vi "FlatToRichnixnet_grpc_CreateSessionRequest.vi"(5 "OutputClusterType":T1, 11 "InputCluster":T3) -> (3 "OutputCluster":T1)   [LabVIEW 2025, in "grpc-xnet_client.lvlib"]
uses:
  nixnet_grpc_CreateSessionRequest_Flat.ctl
  nixnet_grpc_CreateSessionMode.ctl
  nidevice_grpc_SessionInitializationBehavior.ctl
  nixnet_grpc_CreateSessionRequest.ctl
  nixnet_grpc_CreateSessionRequest_mode_enum/nixnet_grpc_CreateSessionRequest_mode_enum.lvclass
  grpc-xnet_client.lvlib
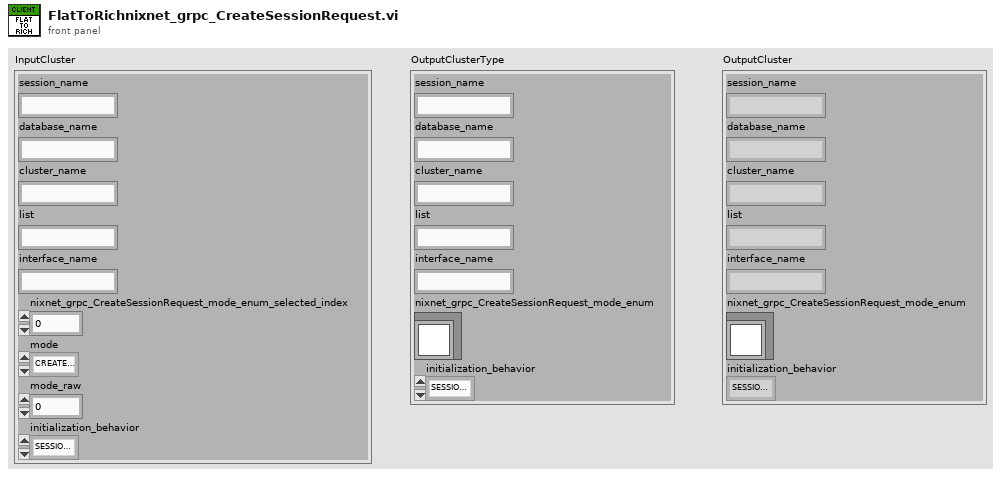
[diagram p1: front panel]
types:
  T1 = typedef "grpc-xnet_client.lvlib/nixnet_grpc_CreateSessionRequest.ctl" = cluster{"session_name":string, "database_name":string, "cluster_name":string, "list":string, "interface_name":string, "nixnet_grpc_CreateSessionRequest_mode_enum":refnum<class "nixnet_grpc_CreateSessionRequest_mode_enum.lvclass">, "initialization_behavior":T2}
  T2 = typedef "grpc-xnet_client.lvlib/nidevice_grpc_SessionInitializationBehavior.ctl" = enum32{"SESSION_INITIALIZATION_BEHAVIOR_UNSPECIFIED", "SESSION_INITIALIZATION_BEHAVIOR_INITIALIZE_NEW", "SESSION_INITIALIZATION_BEHAVIOR_ATTACH_TO_EXISTING"}
  T3 = typedef "grpc-xnet_client.lvlib/nixnet_grpc_CreateSessionRequest_Flat.ctl" = cluster{"session_name":string, "database_name":string, "cluster_name":string, "list":string, "interface_name":string, "nixnet_grpc_CreateSessionRequest_mode_enum_selected_index":i32, "mode":T4, "mode_raw":u32, "initialization_behavior":T2}
  T4 = typedef "grpc-xnet_client.lvlib/nixnet_grpc_CreateSessionMode.ctl" = enum32{"CREATE_SESSION_MODE_SIGNAL_IN_SINGLE_POINT", "CREATE_SESSION_MODE_SIGNAL_IN_WAVEFORM", "CREATE_SESSION_MODE_SIGNAL_IN_XY", "CREATE_SESSION_MODE_SIGNAL_OUT_SINGLE_POINT", "CREATE_SESSION_MODE_SIGNAL_OUT_WAVEFORM", "CREATE_SESSION_MODE_SIGNAL_OUT_XY", "CREATE_SESSION_MODE_FRAME_IN_STREAM", "CREATE_SESSION_MODE_FRAME_IN_QUEUED", "CREATE_SESSION_MODE_FRAME_IN_SINGLE_POINT", "CREATE_SESSION_MODE_FRAME_OUT_STREAM", "CREATE_SESSION_MODE_FRAME_OUT_QUEUED", "CREATE_SESSION_MODE_FRAME_OUT_SINGLE_POINT", "CREATE_SESSION_MODE_SIGNAL_CONVERSION_SINGLE_POINT"}
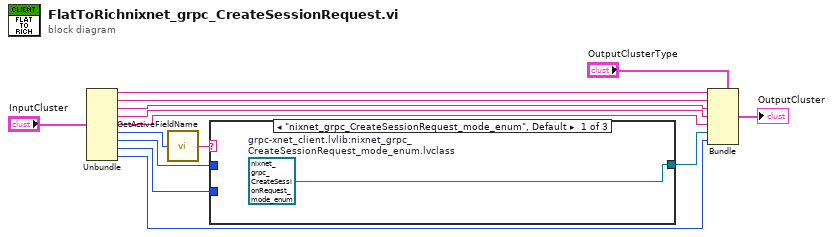
[diagram p0: block diagram]
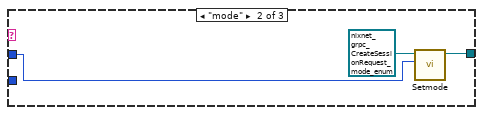
[diagram p2: hidden frame]
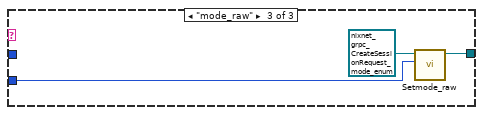
[diagram p3: hidden frame]
diagram:
  n1 = Unbundle "Unbundle"("InputCluster") -> ("session_name"=w11:string, "database_name"=w10:string, "cluster_name"=w9:string, "list"=w8:string, "interface_name"=w7:string, "nixnet_grpc_CreateSessionRequest_mode_enum_selected_index"=w6:i32, "mode"=w3:T4, "mode_raw"=w2:u32, "initialization_behavior"=w1:T2)
  n2 = call "GetActiveFieldName.vi"("protobuf index"=w6) -> ("oneof field name"=w5:string)
  n3 = case "nixnet_grpc_CreateSessionRequest_mode_enum" shown="\"nixnet_grpc_CreateSessionRequest_mode_enum\", Default" w5 {
    tunnel: [w15 w17 w20] -> w4
    tunnel: w3 -> [_ w18 _]
    tunnel: w2 -> [_ _ w21]
    frame "nixnet_grpc_CreateSessionRequest_mode_enum", Default {
      w15 = refnum<class "nixnet_grpc_CreateSessionRequest_mode_enum.lvclass"> refnum  # grpc-xnet_client.lvlib:nixnet_grpc_CreateSessionRequest_mode_enum.lvclass
    }
    frame "mode" {
      n4 = call "Setmode.vi"("Set_Val"=w18, "OneOfTemplate in"=refnum<class "nixnet_grpc_CreateSessionRequest_mode_enum.lvclass"> refnum) -> ("OneOfTemplate out"=w17:refnum<class "nixnet_grpc_CreateSessionRequest_mode_enum.lvclass">)  [unwired: 8 in, 1 out]
    }
    frame "mode_raw" {
      n5 = call "Setmode_raw.vi"("Set_Val"=w21, "OneOfTemplate in"=refnum<class "nixnet_grpc_CreateSessionRequest_mode_enum.lvclass"> refnum) -> ("OneOfTemplate out"=w20:refnum<class "nixnet_grpc_CreateSessionRequest_mode_enum.lvclass">)  [unwired: 8 in, 1 out]
    }
  }
  n6 = Bundle "Bundle"(cluster="OutputClusterType", "session_name"=w11, "database_name"=w10, "cluster_name"=w9, "list"=w8, "interface_name"=w7, "nixnet_grpc_CreateSessionRequest_mode_enum"=w4, "initialization_behavior"=w1) -> (→"OutputCluster":T1)
